vi "Set Cursor Busy State.vi"(8 "Error In":errorcluster, 10 "Busy?":bool, 11 "Splitter Settings UI in":refnum<class "Splitter Settings UI.lvclass">) -> (0 "Error Out":errorcluster, 3 "Splitter Settings UI out":refnum<class "Splitter Settings UI.lvclass">)   [LabVIEW 2017, in "Splitter Settings UI.lvlib" / "Splitter Settings UI.lvclass"]
uses:
  Splitter Settings UI.lvclass
  C:/Program Files (x86)/National Instruments/LabVIEW 2017/vi.lib/MNProjects/Panel Manager/panel-actors/Source/Panel Actor/Panel Actor.lvclass
  <vilib>/MNProjects/Panel Manager/panel-manager/Source/Cursor/Cursor.lvclass
  Splitter Settings UI.lvclass/Splitter Settings UI.ctl
  Splitter Settings UI Messages/Set Cursor Busy State Msg/Set Cursor Busy State Msg.lvclass
  <vilib>/MNProjects/Panel Manager/panel-actors/Source/Panel Actor/Panel Actor.lvclass
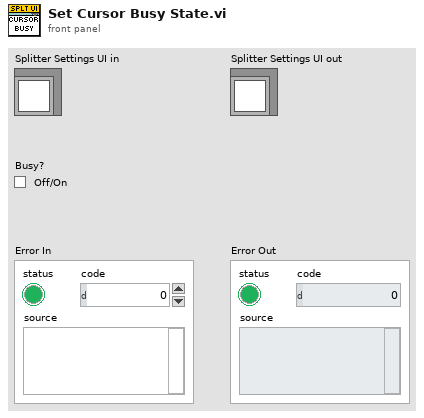
[diagram p1: front panel]
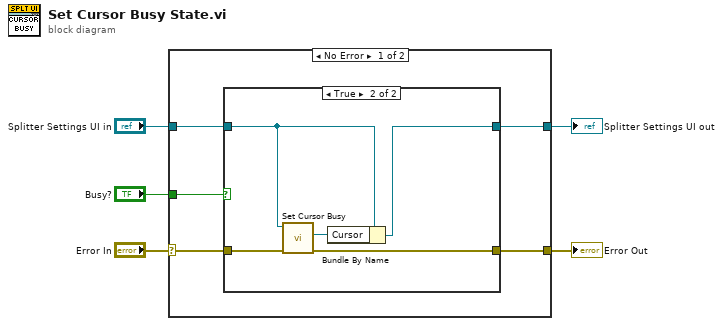
[diagram p0: block diagram]
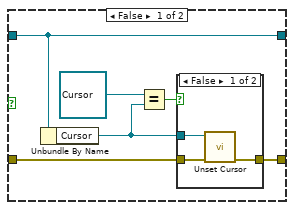
[diagram p2: hidden frame]
diagram:
  n1 = case shown="No Error" "Error In" {
    selector: "Error In" -> [w10 w27]
    tunnel: [w9 w27] -> w2
    tunnel: [w8 w26] -> w4
    tunnel: "Splitter Settings UI in" -> [w7 w26]
    tunnel: "Busy?" -> [w6 _]
    frame No Error {
      n2 = case shown="True" w6 {
        tunnel: w10 -> [w16 w24]
        tunnel: [w15 w22] -> w9
        tunnel: [w14 w21] -> w8
        tunnel: w7 -> [w14 w25]
        frame False {
          n3 = Unbundle By Name(w14) -> ("Cursor"=w13:refnum<class "Cursor.lvclass">)
          n4 = Equal?(x=refnum<class "Cursor.lvclass"> refnum ("MGI-Panel Manager.lvlib:Cursor.lvclass"), y=w13) -> (x = y?=w12:bool)
          n5 = case shown="False" w12 {
            tunnel: w16 -> [w18 w20]
            tunnel: [w17 w20] -> w15
            tunnel: w13 -> [w19 _]
            frame False {
              n6 = call <vilib>:"Unset Cursor.vi"("error in (no error)"=w18, "Cursor in"=w19) -> ("error out"=w17:errorcluster)  [unwired: 9 in]
            }
            frame True {
            }
          }
        }
        frame True {
          (unwired) refnum<class "Set Cursor Busy State Msg.lvclass"> refnum ("Splitter Settings UI.lvlib:Set Cursor Busy State Msg.lvclass")
          n7 = call <vilib>:"Set Cursor Busy.vi"("error in (no error)"=w24, "Panel Actor in"=w25) -> ("error out"=w22:errorcluster, "Cursor"=w23:refnum<class "Cursor.lvclass">)  [unwired: 8 in]
          n8 = Bundle By Name(cluster=w25, "Cursor"=w23) -> (w21:refnum<class "Splitter Settings UI.lvclass">)
        }
      }
    }
    frame Error {
    }
  }
  "Splitter Settings UI out" <- w4
  "Error Out" <- w2
